vi "ROS_Publish.vi"() -> ()   [LabVIEW 2019]
uses:
  C:/Users/Hovhannes/Downloads/ROS.NET-master/ROS.NET-master/ROSPublisherClass/bin/Debug/ROSPublisherClass.dll
  Downloads/ROS.NET-master/ROS.NET-master/ROSPublisherClass/bin/Debug/ROSPublisherClass.dll
panel:
  out "Numeric":i32
  out "error out":errorcluster
  in  "stop":bool
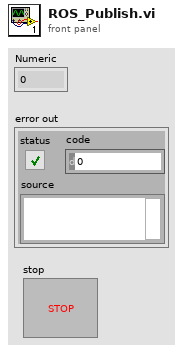
[diagram p1: front panel]
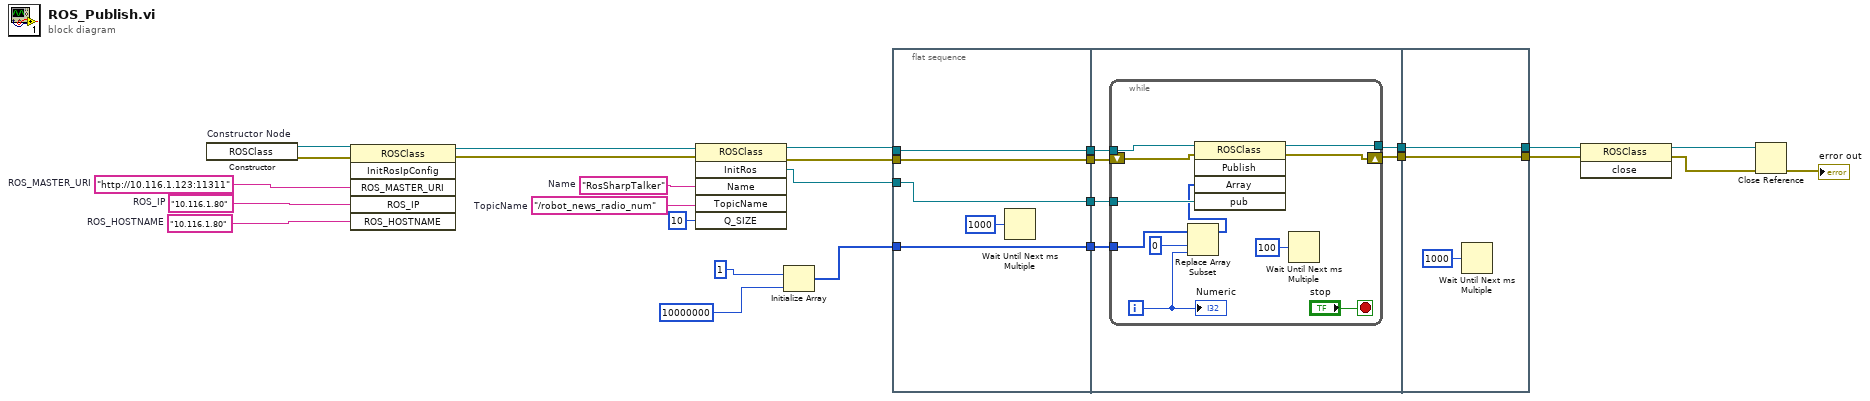
[diagram p0: block diagram]
diagram:
  w2 = "/robot_news_radio_num"  # TopicName
  w3 = "RosSharpTalker"  # Name
  w4 = "10.116.1.80"  # ROS_HOSTNAME
  w6 = "http://10.116.1.123:11311"  # ROS_MASTER_URI
  w5 = "10.116.1.80"  # ROS_IP
  n1 = constructor on="Constructor Node" class="ROSClass"() -> (reference out=w23:refnum<k24>, error out=w12:errorcluster)  [unwired: 3 in, 1 out]
  n2 = invoke class="ROSClass" method="InitRosIpConfig"(reference=w23, error in=w12, "ROS_MASTER_URI"=w6, "ROS_IP"=w5, "ROS_HOSTNAME"=w4) -> (reference out=w11:refnum<k24>, error out=w10:errorcluster)  [unwired: 1 in, 4 out]
  n3 = invoke class="ROSClass" method="InitRos"(reference=w11, error in=w10, "Name"=w3, "TopicName"=w2, "Q_SIZE"=10) -> (reference out=w8:refnum<k24>, error out=w9:errorcluster, "InitRos"=w7:refnum<k24>)  [unwired: 1 in, 3 out]
  n4 = Initialize Array(u8 1, 10000000 ("dimension size")) -> (w18:u8[])
  n5 = flat-sequence {
    tunnel: w9 -> [w31]
    tunnel: w8 -> [w32]
    tunnel: [w32] -> w25
    tunnel: [w31] -> w24
    tunnel: w7 -> [w29]
    tunnel: [w29] -> w22
    tunnel: [w28] -> w19
    tunnel: w18 -> [w28]
    tunnel: w25 -> [w38]
    tunnel: w24 -> [w37]
    tunnel: w22 -> [w34]
    tunnel: w19 -> [w33]
    tunnel: [w36] -> w14
    tunnel: [w35] -> w13
    tunnel: [w51] -> w26
    tunnel: [w52] -> w27
    tunnel: w14 -> [w52]
    tunnel: w13 -> [w51]
    frame #0 {
      n6 = Wait Until Next ms Multiple(millisecond multiple=u32 1000) -> ()  [unwired: 1 out]
    }
    frame #1 {
      n7 = while {
        tunnel: w38 -> [w48]
        tunnel: [w47] -> w36
        shift-right: [w44] -> w35
        shift-left: w37 -> [w45]
        tunnel: w34 -> [w46]
        tunnel: w33 -> [w42]
        i -> [w41]
        stop <- "stop" stop-if-true
        n8 = Replace Array Subset(array=w42, new element=w41, index=0) -> (w39:u8[])
        n9 = invoke class="ROSClass" method="Publish"(reference=w48, error in=w45, "Array"=w39, "pub"=w46) -> (reference out=w47:refnum<k24>, error out=w44:errorcluster)  [unwired: 1 in, 3 out]
        n10 = Wait Until Next ms Multiple(millisecond multiple=u32 100) -> ()  [unwired: 1 out]
        "Numeric" <- w41
      }
    }
    frame #2 {
      n11 = Wait Until Next ms Multiple(millisecond multiple=u32 1000) -> ()  [unwired: 1 out]
    }
  }
  n12 = invoke class="ROSClass" method="close"(reference=w27, error in=w26) -> (reference out=w17:refnum<k24>, error out=w16:errorcluster)  [unwired: 1 in, 1 out]
  n13 = Close Reference(reference=w17, error in (no error)=w16) -> (error out=→"error out":errorcluster)
